vi "FPGA_UtilitiesRead LED.vi"(8 "error in (no error)":errorcluster) -> (0 "error out":errorcluster, 3 "FPGA LED":bool)   [LabVIEW 2017]
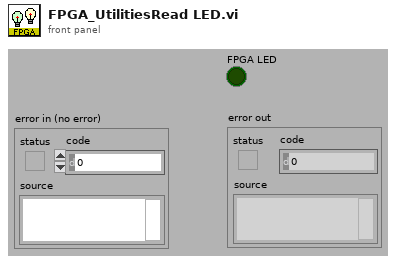
[diagram p1: front panel]
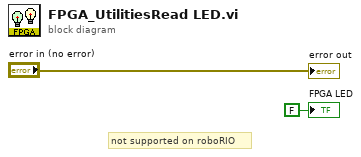
[diagram p0: block diagram]
diagram:
  # "not supported on roboRIO"
  "FPGA LED" <- FALSE ("FPGA LED")
  "error out" <- "error in (no error)"
